vi "Configure Crest Factor Element.vi"(8 "error in (no error)":errorcluster, 9 "Crest Factor (3: CF3)":i32(ring)=3 items=["CF3"=3, "CF6"=6], 11 "VISA resource name":refnum<visa-resource-name>) -> (0 "error out":errorcluster, 3 "VISA resource name out":refnum<visa-resource-name>)   [LabVIEW 2016, in "Yokogawa WT300 Series.lvlib"]
doc: "Configures the Crest Factor element features."
uses:
  Yokogawa WT300 Series.lvlib
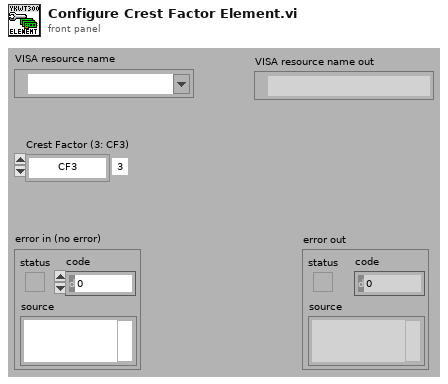
[diagram p1: front panel]
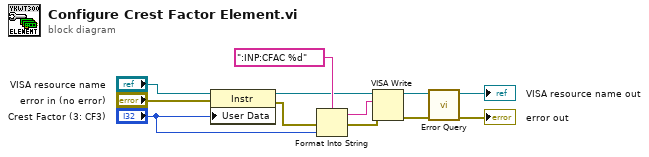
[diagram p0: block diagram]
diagram:
  n1 = property class="Instr"(reference="VISA resource name", error in="error in (no error)", "User Data"="Crest Factor (3: CF3)") -> (reference out=w5:refnum<visa-resource-name>, error out=w3:errorcluster)
  n2 = Format Into String(format string=":INP:CFAC %d" ("Œ`Ž®•¶Žš—ñ"), error in=w3, "Crest Factor (3: CF3)") -> (resulting string=w1:string, error out=w7:errorcluster)  [unwired: 1 in]
  n3 = VISA Write ("VISA書き込み")(VISA resource name=w5, write buffer=w1, error in (no error)=w7) -> (VISA resource name out=w12:refnum<visa-resource-name>, error out=w11:errorcluster)  [unwired: 1 out]
  n4 = call "Error Query.vi"("error in (no error)"=w11, "VISA resource name"=w12) -> ("error out"=→"error out":errorcluster, "VISA resource name out"=→"VISA resource name out":refnum<visa-resource-name>)  [unwired: 6 in, 2 out]
